vi "Discover USB-RF Switch.vi"(8 "error in (no error)":errorcluster) -> (0 "error out":errorcluster, 1 "SER NO.":string, 2 "USB-6501 Present?":bool, 3 "Active Device":tag)   [LabVIEW 2018]
uses:
  <resource>/objmgr/daqmx.rc
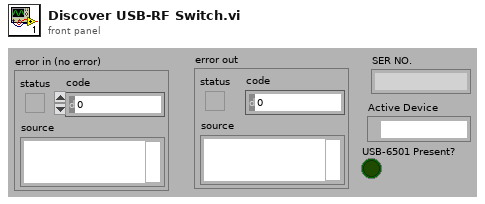
[diagram p1: front panel]
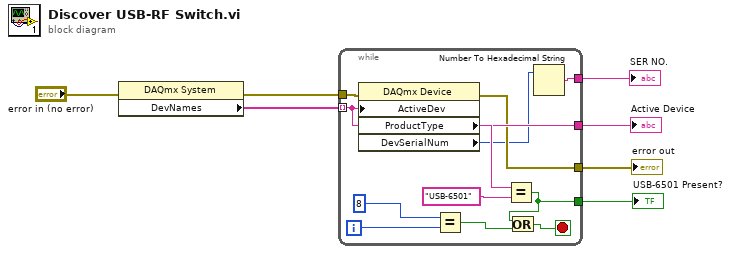
[diagram p0: block diagram]
diagram:
  n1 = property class="DAQmx System"(error in="error in (no error)") -> (error out=w6:errorcluster, "DevNames"=w7:tag[])  [unwired: 1 in, 1 out]
  n2 = while {
    tunnel: w7 -> [w17] mode=indexing
    tunnel: [w17] -> w2
    tunnel: [w13] -> w4
    tunnel: w6 -> [w12]
    tunnel: [w10] -> w3
    tunnel: [w8] -> w5
    i -> [w16]
    stop <- w11 stop-if-true
    n3 = property class="DAQmx Device"(error in=w12, "ActiveDev"=w17) -> (error out=w13:errorcluster, "ProductType"=w19:string, "DevSerialNum"=w9:u32)  [unwired: 1 in, 1 out]
    n4 = Equal?(x=8, y=w16) -> (x = y?=w14:bool)
    n5 = Equal?(x=w19, y="USB-6501") -> (x = y?=w10:bool)
    n6 = Or(x=w10, y=w14) -> (x .or. y?=w11:bool)
    n7 = Number To Hexadecimal String(2:w9) -> (0:w8:string)  [unwired: 1 in]
  }
  "error out" <- w4
  "SER NO." <- w5
  "USB-6501 Present?" <- w3
  "Active Device" <- w2
